vi "Pcre2LibError.vi"(9 "error in":errorcluster, 10 "ErrorCode":i32) -> (1 "error out":errorcluster)   [LabVIEW 2021, in "libpcre2-8.lvlib"]
uses:
  libpcre2-8.lvlib
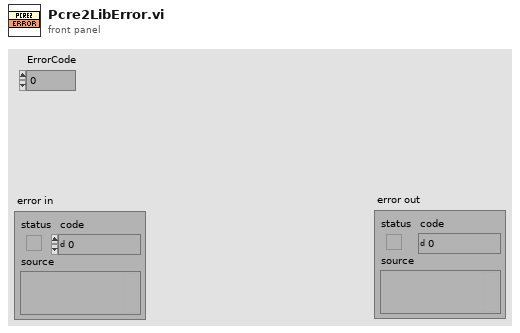
[diagram p1: front panel]
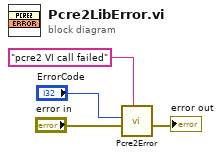
[diagram p0: block diagram]
diagram:
  n1 = call "Pcre2Error.vi"("message"="pcre2 VI call failed", "error in"="error in", "ErrorCode"="ErrorCode") -> ("error out"=→"error out":errorcluster)  [unwired: 8 in]
